vi "LEIN to 485.vi"(0 "LEIN Variation":T1, 7 "CMD":T2={"SID"=0, "ANF"=FALSE, "CMD"=enum."TASK", "DATA"=[]}, 11 "error in (no error)":errorcluster) -> (2 "Header":u16, 3 "Data":u8[](array[numeric]), 6 "Transmitt string":string, 8 "Data  header and CRC":u8[](array[numeric]), 13 "CCITT crc 16":u16, 14 "Data Length":u32, 15 "error out":errorcluster)   [LabVIEW 2011]
uses:
  Defenitions/LEIN CMD Cluster.ctl
  Defenitions/LEIN CMD List.ctl
  Defenitions/LEIN Structure variations.ctl
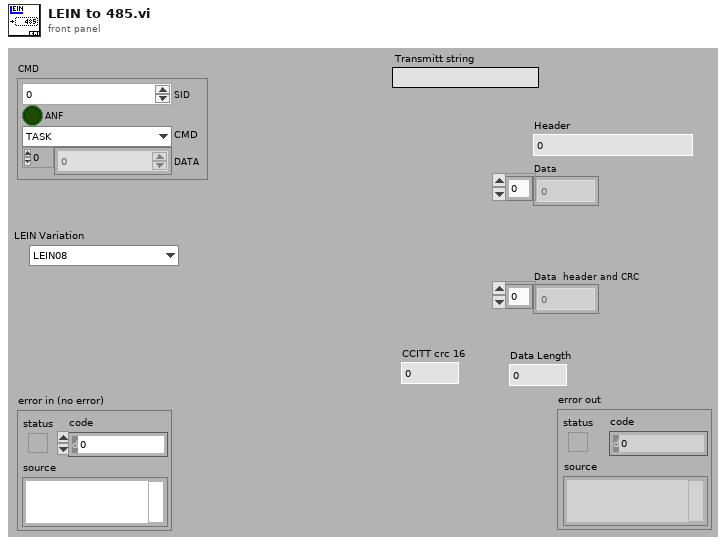
[diagram p1: front panel]
types:
  T1 = typedef "LEIN Structure variations.ctl" = enum16{"LEIN08", "LEIN31", "LEIN63"}
  T2 = typedef "LEIN CMD Cluster.ctl" = cluster{"SID":u8, "ANF":bool, "CMD":T3, "DATA":u8[]}
  T3 = typedef "LEIN CMD List.ctl" = enum8{"ACTI", "TASK", "RES0", "STAT", "RES1", "RES2", "RES3", "USER"}
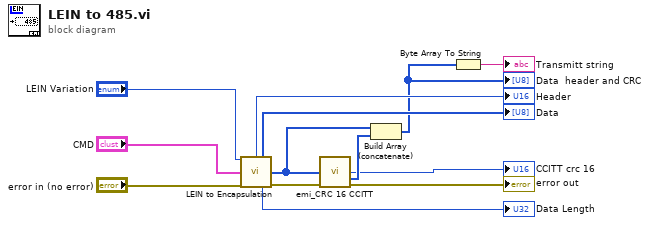
[diagram p0: block diagram]
diagram:
  n1 = call "LEIN to Encapsulation.vi"("LEIN Variation"="LEIN Variation", "CMD"="CMD", "error in (no error)"="error in (no error)") -> ("Header"=→"Header":u16, "Data"=→"Data":u8[], "Data and header"=w5:u8[], "Data Length"=→"Data Length":u32, "error out"=→"error out":errorcluster)  [unwired: 8 in]
  n2 = call "emi_CRC 16 CCITT.vi"("Raw data"=w5) -> ("CCITT crc 16"=→"CCITT crc 16":u16, "CCITT crc 16 bytes"=w4:u8[])  [unwired: 13 in]
  n3 = Build Array (concatenate)(w5, w4) -> (w2:u8[])
  "Data  header and CRC" <- w2
  n4 = Byte Array To String(unsigned byte array=w2) -> (string=→"Transmitt string":string)
